vi "Impulso.vi"(2 "appended array":dbl[](array[numeric])) -> (0 "Parametros":cluster{i32, i32, i32, i32, i32, dbl})   [LabVIEW 2014]
panel:
  in  "Reset":bool
  in  "Start":bool
  out "Ganancia del Impulso":dbl
  in  "Remove Button 6":bool
  in  "Add Button 6":bool
  out "Profundidad del Impulso":i32
  in  "Remove Button 5":bool
  in  "Add Button 5":bool
  out "Frecuencia del Impulso":i32
  in  "Remove Button 4":bool
  in  "Add Button 4":bool
  out "Longitud de Ruptura":i32
  in  "Remove Button 3":bool
  in  "Add Button 3":bool
  out "Longitud Impulso":i32
  in  "Remove Button 2":bool
  in  "Add Button 2":bool
  out "Tiempo del Programa":i32
  in  "Remove Button":bool
  in  "Add Button":bool
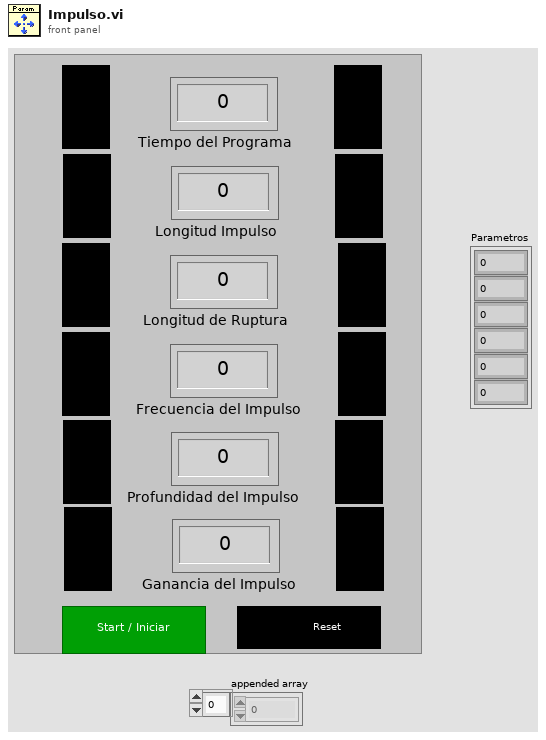
[diagram p1: front panel]
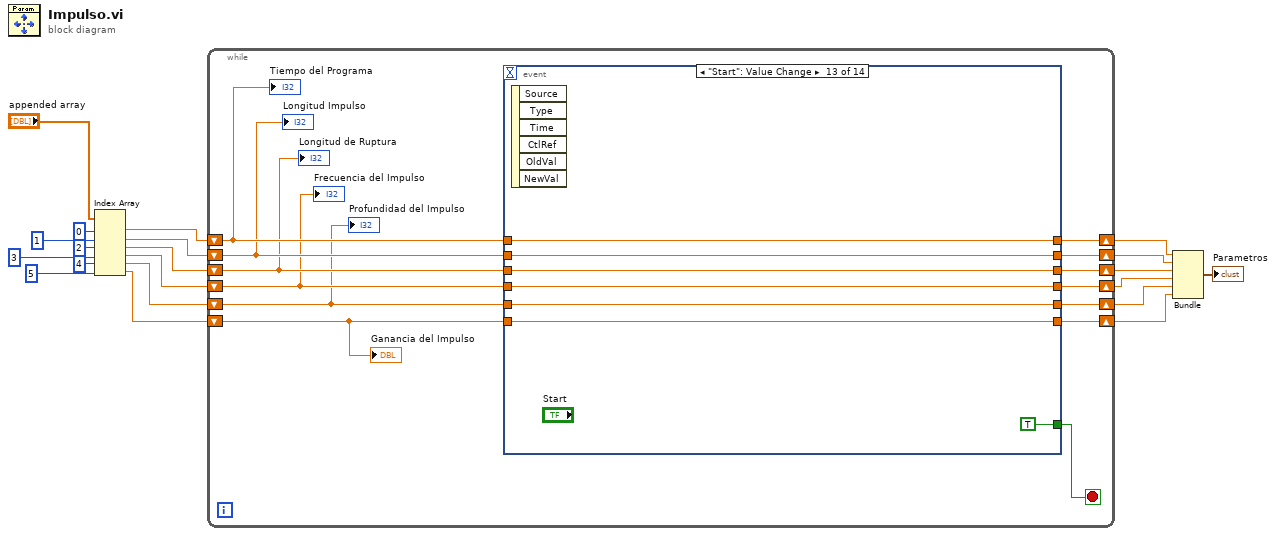
[diagram p0: block diagram]
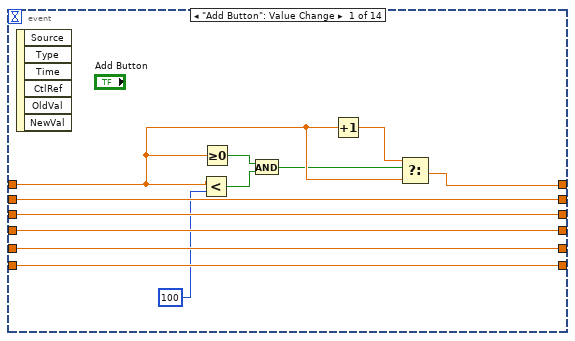
[diagram p2: hidden frame]
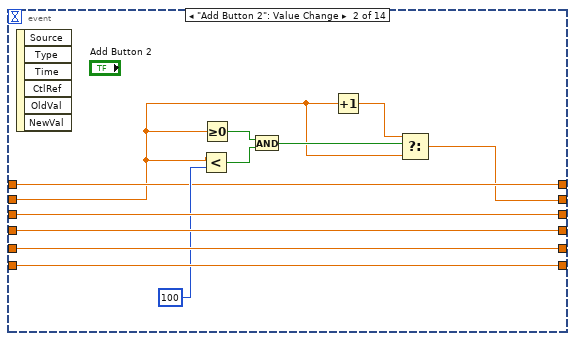
[diagram p3: hidden frame]
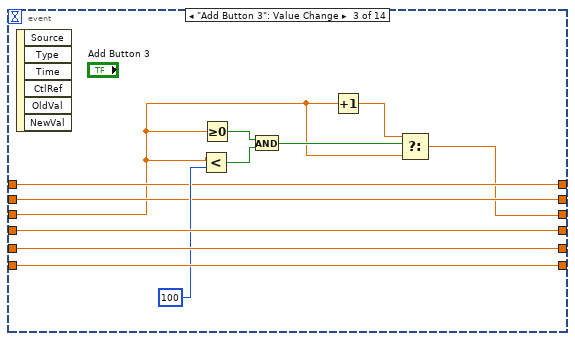
[diagram p4: hidden frame]
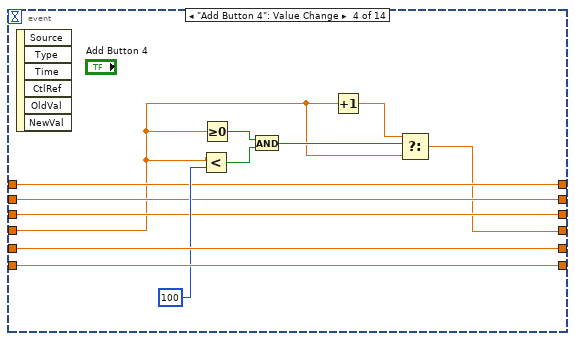
[diagram p5: hidden frame]
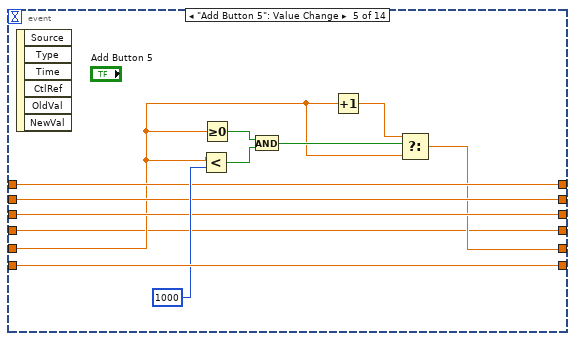
[diagram p6: hidden frame]
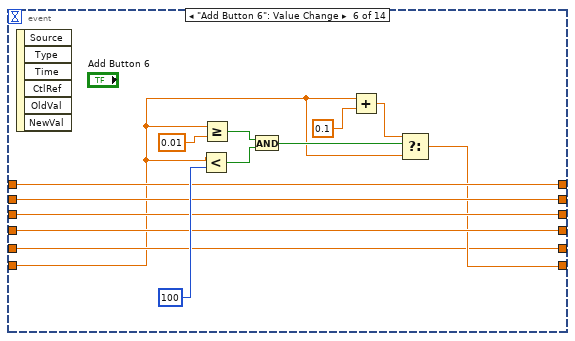
[diagram p7: hidden frame]
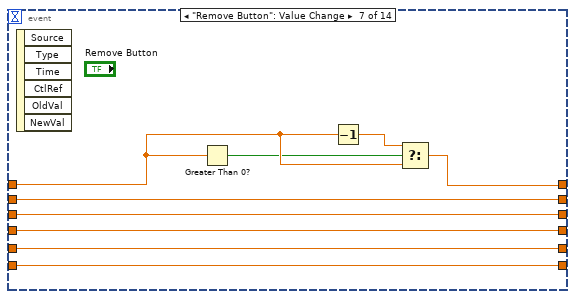
[diagram p8: hidden frame]
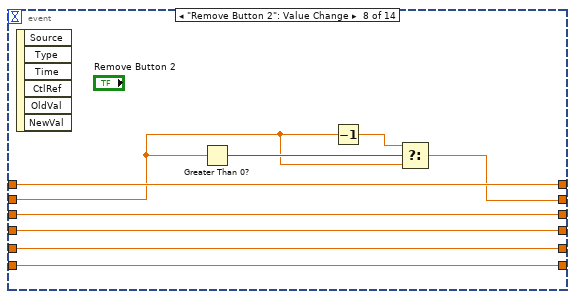
[diagram p9: hidden frame]
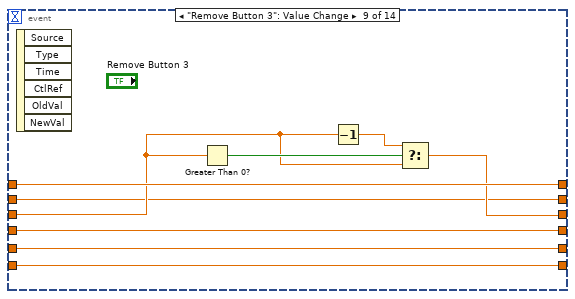
[diagram p10: hidden frame]
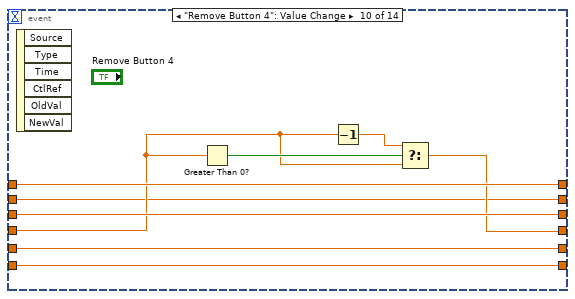
[diagram p11: hidden frame]
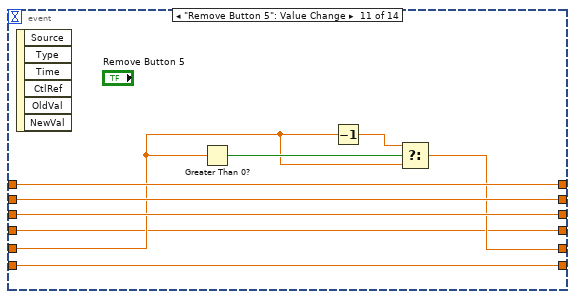
[diagram p12: hidden frame]
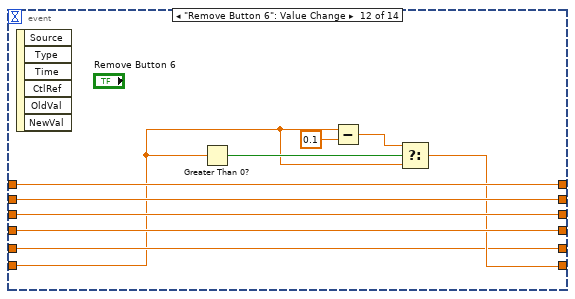
[diagram p13: hidden frame]
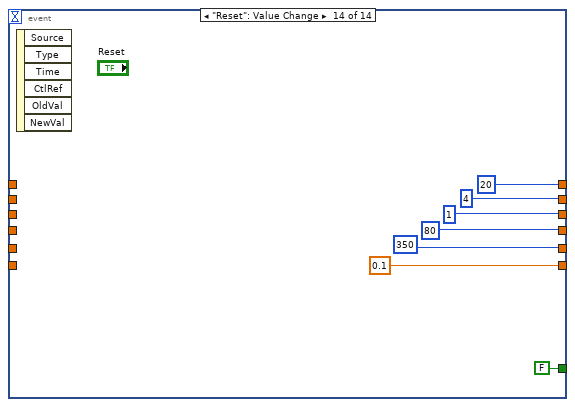
[diagram p14: hidden frame]
diagram:
  n1 = Index Array(array="appended array", index #1=0 ("index"), index #2=1 ("index"), index #3=2 ("index"), index #4=3 ("index"), index #5=4 ("index"), index #6=5 ("index")) -> (element #1=w11:dbl, element #2=w9:dbl, element #3=w7:dbl, element #4=w4:dbl, element #5=w2:dbl, element #6=w1:dbl)
  n2 = while {
    shift-right: [w32] -> w20
    shift-left: w11 -> [w26]
    shift-right: [w31] -> w17
    shift-left: w9 -> [w25]
    shift-right: [w30] -> w19
    shift-left: w7 -> [w24]
    shift-right: [w29] -> w18
    shift-left: w4 -> [w23]
    shift-right: [w28] -> w16
    shift-left: w2 -> [w22]
    shift-right: [w27] -> w15
    shift-left: w1 -> [w21]
    stop <- w33 stop-if-true
    n3 = event shown="[12] \"Start\": Value Change" {
      selector: _ -> [_ _ _ _ _ _ _ _ _ _ _ _ _ _]
      dyn-events: _ -> [_ _ _ _ _ _ _ _ _ _ _ _ _ _]
      timeout: _ -> [_ _ _ _ _ _ _ _ _ _ _ _ _ _]
      tunnel: w26 -> [w45 w48 w61 w74 w87 w102 w116 w119 w129 w138 w148 w159 w163 _]
      tunnel: w25 -> [w43 w46 w60 w73 w86 w101 w114 w117 w126 w135 w147 w158 w164 _]
      tunnel: w24 -> [w42 w57 w58 w72 w85 w100 w113 w125 w128 w143 w152 w162 w165 _]
      tunnel: w23 -> [w41 w56 w69 w70 w82 w99 w112 w124 w134 w136 w144 w157 w166 _]
      tunnel: w22 -> [w40 w55 w68 w81 w84 w97 w111 w123 w133 w142 w146 w155 w167 _]
      tunnel: w21 -> [w39 w54 w67 w80 w93 w95 w110 w122 w132 w141 w151 w154 w168 _]
      tunnel: [w44 w48 w61 w74 w87 w102 w115 w119 w129 w138 w148 w159 w163 20] -> w32
      tunnel: [w43 w47 w60 w73 w86 w101 w114 w118 w126 w135 w147 w158 w164 4] -> w31
      tunnel: [w42 w57 w59 w72 w85 w100 w113 w125 w127 w143 w152 w162 w165 1] -> w30
      tunnel: [w41 w56 w69 w71 w82 w99 w112 w124 w134 w137 w144 w157 w166 80] -> w29
      tunnel: [w40 w55 w68 w81 w83 w97 w111 w123 w133 w142 w145 w155 w167 350] -> w28
      tunnel: [w39 w54 w67 w80 w93 w98 w110 w122 w132 w141 w151 w156 w168 0.1] -> w27
      tunnel: [_ _ _ _ _ _ _ _ _ _ _ _ TRUE FALSE] -> w33
      event "Add Button": Value Change {
        n4 = event-data() -> ()  [unwired: 1 in, 6 out]
        n5 = Less?(x=w45, y=100) -> (x < y?=w37:bool)
        n6 = Greater Or Equal To 0?(x=w45) -> (x >= 0?=w38:bool)
        n7 = And(x=w38, y=w37) -> (x .and. y?=w35:bool)
        n8 = Increment(x=w45) -> (x+1=w34:dbl)
        n9 = Select(t=w34, s=w35, f=w45) -> (s? t:f=w44:dbl)
      }
      event "Add Button 2": Value Change {
        n10 = event-data() -> ()  [unwired: 1 in, 6 out]
        n11 = Less?(x=w46, y=100) -> (x < y?=w52:bool)
        n12 = Greater Or Equal To 0?(x=w46) -> (x >= 0?=w53:bool)
        n13 = And(x=w53, y=w52) -> (x .and. y?=w50:bool)
        n14 = Increment(x=w46) -> (x+1=w49:dbl)
        n15 = Select(t=w49, s=w50, f=w46) -> (s? t:f=w47:dbl)
      }
      event "Add Button 3": Value Change {
        n16 = event-data() -> ()  [unwired: 1 in, 6 out]
        n17 = Less?(x=w58, y=100) -> (x < y?=w65:bool)
        n18 = Greater Or Equal To 0?(x=w58) -> (x >= 0?=w66:bool)
        n19 = And(x=w66, y=w65) -> (x .and. y?=w63:bool)
        n20 = Increment(x=w58) -> (x+1=w62:dbl)
        n21 = Select(t=w62, s=w63, f=w58) -> (s? t:f=w59:dbl)
      }
      event "Add Button 4": Value Change {
        n22 = event-data() -> ()  [unwired: 1 in, 6 out]
        n23 = Less?(x=w70, y=100) -> (x < y?=w78:bool)
        n24 = Greater Or Equal To 0?(x=w70) -> (x >= 0?=w79:bool)
        n25 = And(x=w79, y=w78) -> (x .and. y?=w76:bool)
        n26 = Increment(x=w70) -> (x+1=w75:dbl)
        n27 = Select(t=w75, s=w76, f=w70) -> (s? t:f=w71:dbl)
      }
      event "Add Button 5": Value Change {
        n28 = event-data() -> ()  [unwired: 1 in, 6 out]
        n29 = Less?(x=w84, y=1000) -> (x < y?=w91:bool)
        n30 = Greater Or Equal To 0?(x=w84) -> (x >= 0?=w92:bool)
        n31 = And(x=w92, y=w91) -> (x .and. y?=w89:bool)
        n32 = Increment(x=w84) -> (x+1=w88:dbl)
        n33 = Select(t=w88, s=w89, f=w84) -> (s? t:f=w83:dbl)
      }
      event "Add Button 6": Value Change {
        n34 = event-data() -> ()  [unwired: 1 in, 6 out]
        n35 = Less?(x=w95, y=100) -> (x < y?=w106:bool)
        n36 = Greater Or Equal?(x=w95, y=0.01) -> (x >= y?=w107:bool)
        n37 = And(x=w107, y=w106) -> (x .and. y?=w104:bool)
        n38 = Add(x=w95, y=0.1) -> (x+y=w103:dbl)
        n39 = Select(t=w103, s=w104, f=w95) -> (s? t:f=w98:dbl)
      }
      event "Remove Button": Value Change {
        n40 = event-data() -> ()  [unwired: 1 in, 6 out]
        n41 = Greater Than 0?(x=w116) -> (x > 0?=w108:bool)
        n42 = Decrement(x=w116) -> (x-1=w109:dbl)
        n43 = Select(t=w109, s=w108, f=w116) -> (s? t:f=w115:dbl)
      }
      event "Remove Button 2": Value Change {
        n44 = event-data() -> ()  [unwired: 1 in, 6 out]
        n45 = Greater Than 0?(x=w117) -> (x > 0?=w120:bool)
        n46 = Decrement(x=w117) -> (x-1=w121:dbl)
        n47 = Select(t=w121, s=w120, f=w117) -> (s? t:f=w118:dbl)
      }
      event "Remove Button 3": Value Change {
        n48 = event-data() -> ()  [unwired: 1 in, 6 out]
        n49 = Greater Than 0?(x=w128) -> (x > 0?=w130:bool)
        n50 = Decrement(x=w128) -> (x-1=w131:dbl)
        n51 = Select(t=w131, s=w130, f=w128) -> (s? t:f=w127:dbl)
      }
      event "Remove Button 4": Value Change {
        n52 = event-data() -> ()  [unwired: 1 in, 6 out]
        n53 = Greater Than 0?(x=w136) -> (x > 0?=w139:bool)
        n54 = Decrement(x=w136) -> (x-1=w140:dbl)
        n55 = Select(t=w140, s=w139, f=w136) -> (s? t:f=w137:dbl)
      }
      event "Remove Button 5": Value Change {
        n56 = event-data() -> ()  [unwired: 1 in, 6 out]
        n57 = Greater Than 0?(x=w146) -> (x > 0?=w149:bool)
        n58 = Decrement(x=w146) -> (x-1=w150:dbl)
        n59 = Select(t=w150, s=w149, f=w146) -> (s? t:f=w145:dbl)
      }
      event "Remove Button 6": Value Change {
        n60 = event-data() -> ()  [unwired: 1 in, 6 out]
        n61 = Greater Than 0?(x=w154) -> (x > 0?=w160:bool)
        n62 = Subtract(x=w154, y=0.1) -> (x-y=w161:dbl)
        n63 = Select(t=w161, s=w160, f=w154) -> (s? t:f=w156:dbl)
      }
      event "Start": Value Change {
        n64 = event-data() -> ()  [unwired: 1 in, 6 out]
      }
      event "Reset": Value Change {
        n65 = event-data() -> ()  [unwired: 1 in, 6 out]
      }
    }
    "Tiempo del Programa" <- w26
    "Longitud Impulso" <- w25
    "Longitud de Ruptura" <- w24
    "Frecuencia del Impulso" <- w23
    "Profundidad del Impulso" <- w22
    "Ganancia del Impulso" <- w21
  }
  n66 = Bundle(w20, w17, w19, w18, w16, w15) -> (→"Parametros":cluster{dbl, dbl, dbl, dbl, dbl, dbl})  [unwired: 1 in]
